vi "Start AsyncSum.vi"(8 "error in (no error)":errorcluster, 9 "B":i32, 10 "A":i32, 11 "path in":path) -> (0 "error out":errorcluster, 1 "LVUserEvent CallBack Reference":refnum<user-event>, 2 "Handle":u64, 3 "dup path":path, 4 "AsyncSum Event Register":refnum<event-registration>)   [LabVIEW 2016, in "DemoSkeleton.lvlib"]
uses:
  DemoSkeleton.lvlib
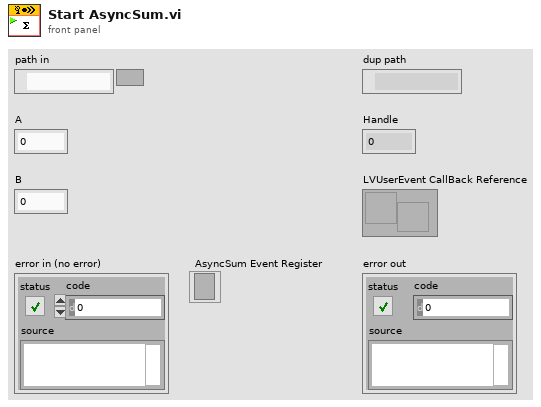
[diagram p1: front panel]
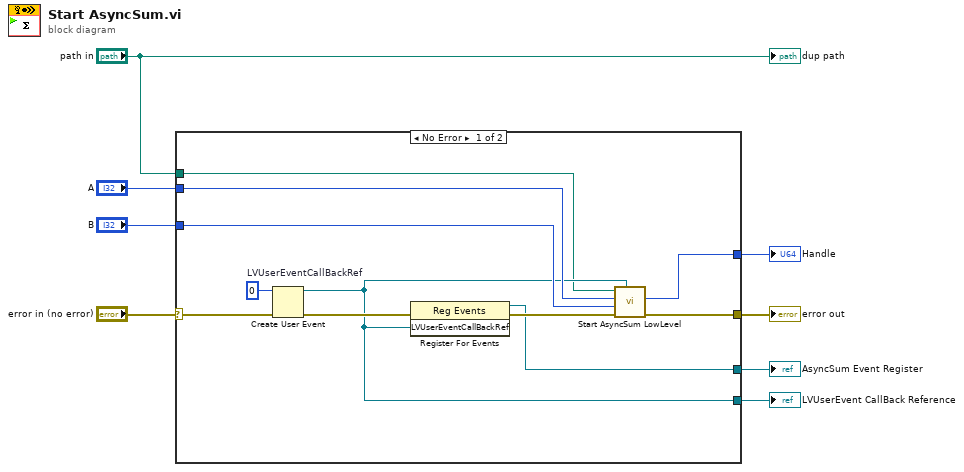
[diagram p0: block diagram]
diagram:
  n1 = case shown="No Error" "error in (no error)" {
    selector: "error in (no error)" -> [w14 w20]
    tunnel: [w10 _] -> w8
    tunnel: "A" -> [w18 _]
    tunnel: "B" -> [w17 _]
    tunnel: [w16 _] -> w5
    tunnel: [w15 w20] -> w4
    tunnel: [w11 _] -> w2
    tunnel: "path in" -> [w9 _]
    frame No Error {
      w19 = i64 0  # LVUserEventCallBackRef
      n2 = Create User Event(user event datatype=w19, error in=w14) -> (user event=w10:refnum<user-event>, error out=w13:errorcluster)
      n3 = register-events(error in=w13, w10) -> (reference out=w11:refnum<event-registration>, error out=w12:errorcluster)  [unwired: 1 in]
      n4 = call "Start AsyncSum LowLevel.vi"("LVUserEventCallBackRef"=w10, "error in"=w12, "B"=w17, "A"=w18, "path in"=w9) -> ("error out"=w15:errorcluster, "Handle"=w16:u64)  [unwired: 4 in, 1 out]
    }
    frame Error {
    }
  }
  "Handle" <- w5
  "error out" <- w4
  "LVUserEvent CallBack Reference" <- w8
  "AsyncSum Event Register" <- w2
  "dup path" <- "path in"
